vi "Move around TRAD v2.vi"() -> ()   [LabVIEW 2014]
uses:
  <vilib>/Instr/_visa.llb/VISA Configure Serial Port (Instr).vi
panel:
  in  "Numeric 2":i32
  in  "Short B desired":dbl
  in  "Short A desired":dbl
  in  "Move to position":bool
  in  "Home":bool
  out "number 2":i32
  out "number":i32
  in  "Dir":bool
  in  "Steps":u16(ring) items=["5", "10", "100", "1000", "10000"]
  in  "Move Tuner":bool
  in  "Save Position":bool
  in  "stop":bool
  in  "GO":bool
  in  "Change What":bool
  in  "Direction":bool
  out "Short B Value":dbl
  out "Short A Value":dbl
  out "Tuner Position":string
  # "Forward"
  # "Magnitude"
  # "Phase\nDifference"
  # "UP"
  # "Backward"
  # "DOWN"
  # "Move to a Particular Position"
  # "Go"
  # "Short B"
  # "Short A"
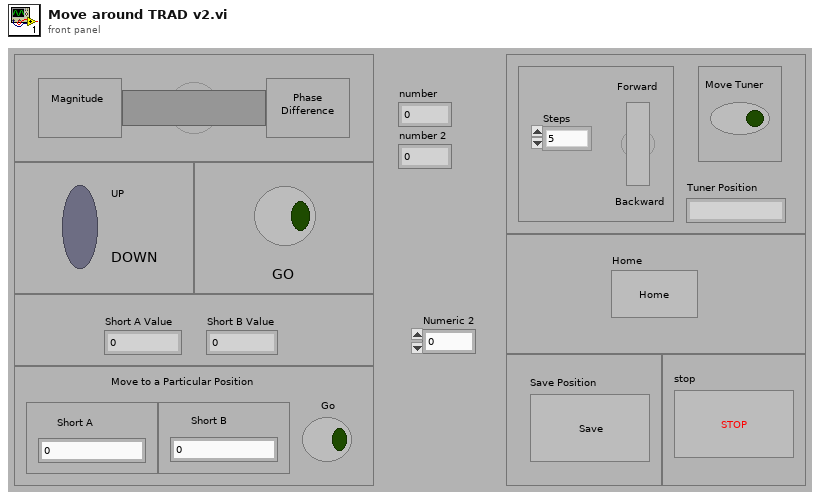
[diagram p1: front panel]
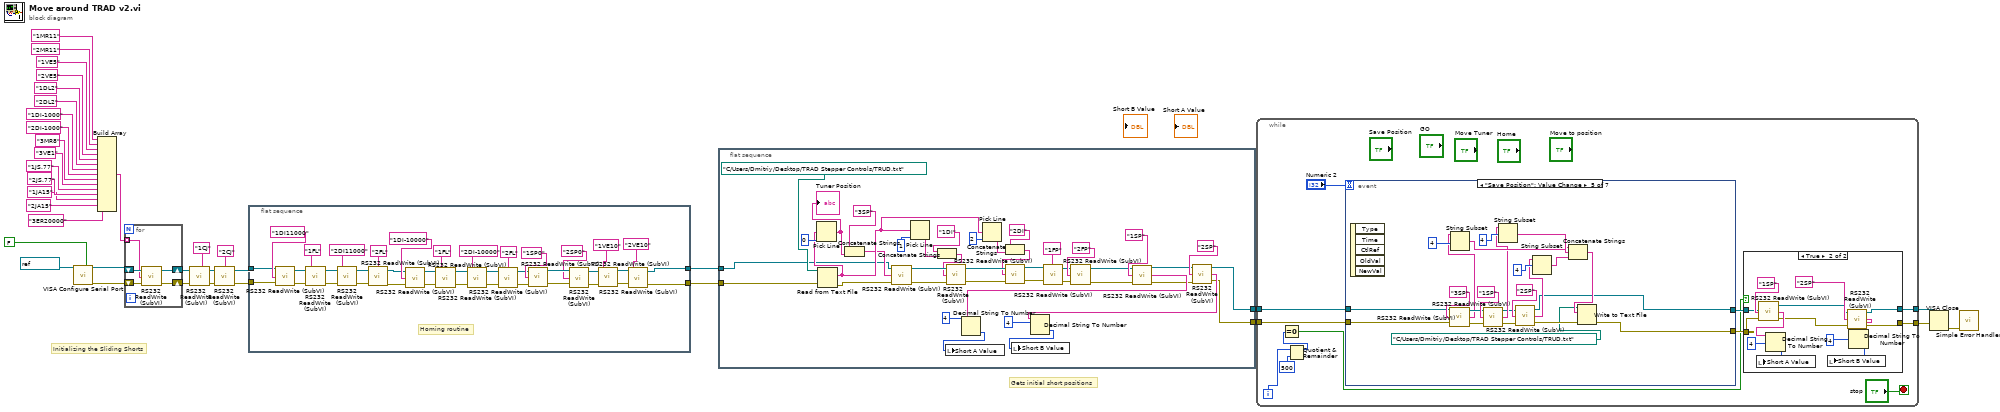
[diagram p0: block diagram]
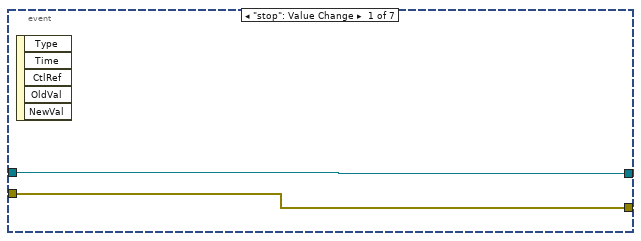
[diagram p3: hidden frame]
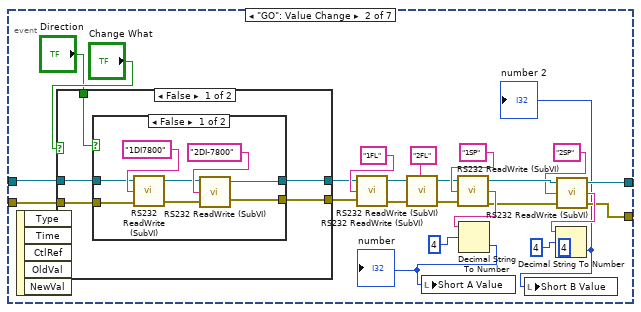
[diagram p4: hidden frame]
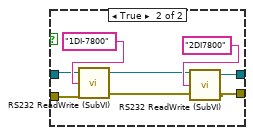
[diagram p5: hidden frame]
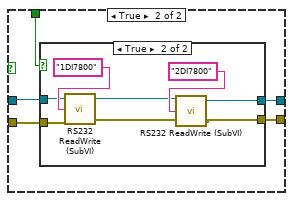
[diagram p6: hidden frame]
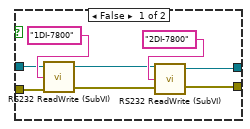
[diagram p7: hidden frame]
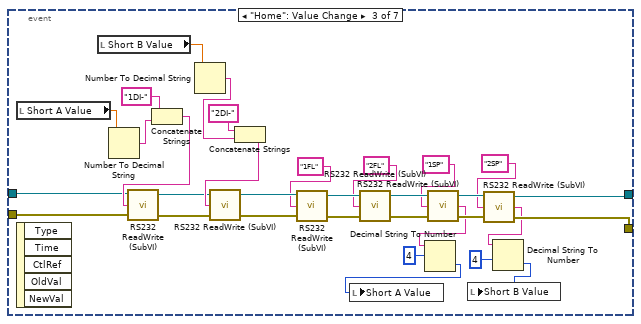
[diagram p8: hidden frame]
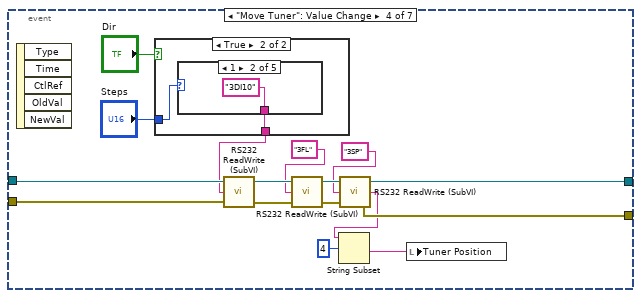
[diagram p9: hidden frame]
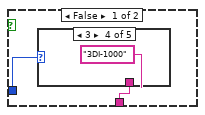
[diagram p10: hidden frame]
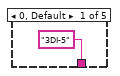
[diagram p11: hidden frame]
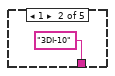
[diagram p12: hidden frame]
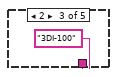
[diagram p13: hidden frame]
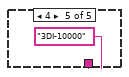
[diagram p14: hidden frame]
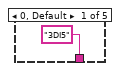
[diagram p15: hidden frame]
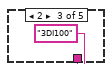
[diagram p16: hidden frame]
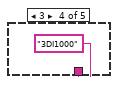
[diagram p17: hidden frame]
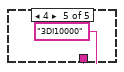
[diagram p18: hidden frame]
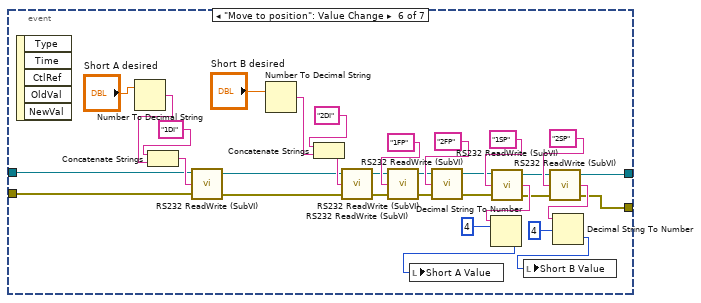
[diagram p19: hidden frame]
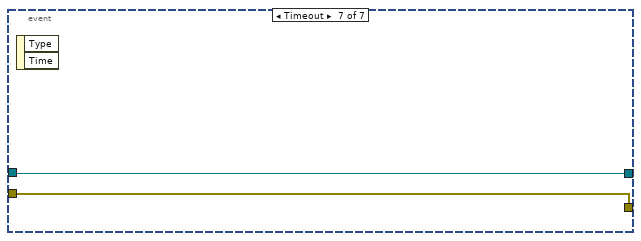
[diagram p20: hidden frame]
diagram:
  # "Initializing the Sliding Shorts"
  # "Gets initial short positions"
  n1 = call-poly "VISA Configure Serial Port"("VISA resource name"=refnum<visa-resource-name> "COM3", "Enable Termination\nChar (T)"=FALSE) -> ("VISA resource name out"=w18:refnum<visa-resource-name>, "error out"=w17:errorcluster)  [unwired: 12 in]
  n2 = Build Array("1MR11" ("Command to send to controller"), "2MR11" ("Command to send to controller"), "1VE5" ("Command to send to controller"), "2VE5" ("Command to send to controller"), "1DL2" ("Command to send to controller"), "2DL2" ("Command to send to controller"), "1DI-1000" ("Command to send to controller"), "2DI-1000" ("Command to send to controller"), "3MR8" ("Command to send to controller"), "3VE1" ("Command to send to controller"), "1JS.77", "2JS.77", "1JA15", "2JA15", "3ER20000") -> (w29:string[])
  n3 = for {
    shift-right: [w38] -> w15
    shift-left: w17 -> [w39]
    shift-right: [w37] -> w16
    shift-left: w18 -> [w40]
    tunnel: w29 -> [w36] mode=indexing
    n4 = call "RS232 ReadWrite (SubVI).vi"("error in (no error)"=w39, "Command to send to controller"=w36, "VISA resource name"=w40) -> ("error out"=w38:errorcluster, "VISA resource name out"=w37:refnum<visa-resource-name>)  [unwired: 1 out]
  }
  n5 = call "RS232 ReadWrite (SubVI).vi"("error in (no error)"=w15, "Command to send to controller"="1CJ", "VISA resource name"=w16) -> ("error out"=w6:errorcluster, "VISA resource name out"=w7:refnum<visa-resource-name>)  [unwired: 1 out]
  n6 = call "RS232 ReadWrite (SubVI).vi"("error in (no error)"=w6, "Command to send to controller"="2CJ", "VISA resource name"=w7) -> ("error out"=w13:errorcluster, "VISA resource name out"=w14:refnum<visa-resource-name>)  [unwired: 1 out]
  n7 = flat-sequence {
    tunnel: w13 -> [w63]
    tunnel: w14 -> [w64]
    tunnel: [w44] -> w4
    tunnel: [w43] -> w3
    frame #0 {
      # "Homing routine"
      n8 = call "RS232 ReadWrite (SubVI).vi"("error in (no error)"=w63, "Command to send to controller"="1DI11000", "VISA resource name"=w64) -> ("error out"=w75:errorcluster, "VISA resource name out"=w76:refnum<visa-resource-name>)  [unwired: 1 out]
      n9 = call "RS232 ReadWrite (SubVI).vi"("error in (no error)"=w75, "Command to send to controller"="1FL", "VISA resource name"=w76) -> ("error out"=w73:errorcluster, "VISA resource name out"=w74:refnum<visa-resource-name>)  [unwired: 1 out]
      n10 = call "RS232 ReadWrite (SubVI).vi"("error in (no error)"=w73, "Command to send to controller"="2DI11000", "VISA resource name"=w74) -> ("error out"=w71:errorcluster, "VISA resource name out"=w72:refnum<visa-resource-name>)  [unwired: 1 out]
      n11 = call "RS232 ReadWrite (SubVI).vi"("error in (no error)"=w71, "Command to send to controller"="2FL", "VISA resource name"=w72) -> ("error out"=w52:errorcluster, "VISA resource name out"=w51:refnum<visa-resource-name>)  [unwired: 1 out]
      n12 = call "RS232 ReadWrite (SubVI).vi"("error in (no error)"=w52, "Command to send to controller"="1DI-10000", "VISA resource name"=w51) -> ("error out"=w61:errorcluster, "VISA resource name out"=w62:refnum<visa-resource-name>)  [unwired: 1 out]
      n13 = call "RS232 ReadWrite (SubVI).vi"("error in (no error)"=w61, "Command to send to controller"="1FL", "VISA resource name"=w62) -> ("error out"=w59:errorcluster, "VISA resource name out"=w60:refnum<visa-resource-name>)  [unwired: 1 out]
      n14 = call "RS232 ReadWrite (SubVI).vi"("error in (no error)"=w59, "Command to send to controller"="2DI-10000", "VISA resource name"=w60) -> ("error out"=w57:errorcluster, "VISA resource name out"=w58:refnum<visa-resource-name>)  [unwired: 1 out]
      n15 = call "RS232 ReadWrite (SubVI).vi"("error in (no error)"=w57, "Command to send to controller"="2FL", "VISA resource name"=w58) -> ("error out"=w49:errorcluster, "VISA resource name out"=w50:refnum<visa-resource-name>)  [unwired: 1 out]
      n16 = call "RS232 ReadWrite (SubVI).vi"("error in (no error)"=w49, "Command to send to controller"="1SP0", "VISA resource name"=w50) -> ("error out"=w77:errorcluster, "VISA resource name out"=w78:refnum<visa-resource-name>)  [unwired: 1 out]
      n17 = call "RS232 ReadWrite (SubVI).vi"("error in (no error)"=w77, "Command to send to controller"="2SP0", "VISA resource name"=w78) -> ("error out"=w47:errorcluster, "VISA resource name out"=w48:refnum<visa-resource-name>)  [unwired: 1 out]
      n18 = call "RS232 ReadWrite (SubVI).vi"("error in (no error)"=w47, "Command to send to controller"="1VE10", "VISA resource name"=w48) -> ("error out"=w45:errorcluster, "VISA resource name out"=w46:refnum<visa-resource-name>)  [unwired: 1 out]
      n19 = call "RS232 ReadWrite (SubVI).vi"("error in (no error)"=w45, "Command to send to controller"="2VE10", "VISA resource name"=w46) -> ("error out"=w43:errorcluster, "VISA resource name out"=w44:refnum<visa-resource-name>)  [unwired: 1 out]
    }
  }
  n20 = flat-sequence {
    tunnel: [w82] -> w34
    tunnel: [w81] -> w2
    tunnel: w3 -> [w117]
    tunnel: w4 -> [w97]
    frame #0 {
      n21 = Read from Text File(file (use dialog)=path "C:/Users/Dmitriy/Desktop/TRAD Stepper Controls/TRUD.txt", error in=w117) -> (text=w115:string, error out=w112:errorcluster)  [unwired: 2 in, 2 out]
      n22 = Pick Line(multi-line string=w115, line index=0) -> (output string=w107:string)  [unwired: 1 in]
      "Tuner Position" <- w107
      n23 = Concatenate Strings("3SP" ("string"), w107) -> (w106:string)
      n24 = call "RS232 ReadWrite (SubVI).vi"("error in (no error)"=w112, "Command to send to controller"=w106, "VISA resource name"=w97) -> ("error out"=w113:errorcluster, "VISA resource name out"=w111:refnum<visa-resource-name>)  [unwired: 1 out]
      n25 = Pick Line(multi-line string=w115, line index=1) -> (output string=w101:string)  [unwired: 1 in]
      n26 = Concatenate Strings("1DI" ("string"), w101) -> (w103:string)
      n27 = call "RS232 ReadWrite (SubVI).vi"("error in (no error)"=w113, "Command to send to controller"=w103, "VISA resource name"=w111) -> ("error out"=w114:errorcluster, "VISA resource name out"=w110:refnum<visa-resource-name>)  [unwired: 1 out]
      n28 = Pick Line(multi-line string=w115, line index=2) -> (output string=w100:string)  [unwired: 1 in]
      n29 = Concatenate Strings("2DI" ("string"), w100) -> (w102:string)
      n30 = call "RS232 ReadWrite (SubVI).vi"("error in (no error)"=w114, "Command to send to controller"=w102, "VISA resource name"=w110) -> ("error out"=w93:errorcluster, "VISA resource name out"=w94:refnum<visa-resource-name>)  [unwired: 1 out]
      n31 = call "RS232 ReadWrite (SubVI).vi"("error in (no error)"=w93, "Command to send to controller"="1FP", "VISA resource name"=w94) -> ("error out"=w95:errorcluster, "VISA resource name out"=w92:refnum<visa-resource-name>)  [unwired: 1 out]
      n32 = call "RS232 ReadWrite (SubVI).vi"("error in (no error)"=w95, "Command to send to controller"="2FP", "VISA resource name"=w92) -> ("error out"=w79:errorcluster, "VISA resource name out"=w80:refnum<visa-resource-name>)  [unwired: 1 out]
      n33 = call "RS232 ReadWrite (SubVI).vi"("error in (no error)"=w79, "Command to send to controller"="1SP", "VISA resource name"=w80) -> ("error out"=w83:errorcluster, "String read from controller"=w87:string, "VISA resource name out"=w84:refnum<visa-resource-name>)
      n34 = Decimal String To Number(string=w87, offset=4) -> (number=w98:i32)  [unwired: 1 in, 1 out]
      n35 = local write "Short A Value"(w98) -> ()
      n36 = call "RS232 ReadWrite (SubVI).vi"("error in (no error)"=w83, "Command to send to controller"="2SP", "VISA resource name"=w84) -> ("error out"=w81:errorcluster, "String read from controller"=w88:string, "VISA resource name out"=w82:refnum<visa-resource-name>)
      n37 = Decimal String To Number(string=w88, offset=4) -> (number=w99:i32)  [unwired: 1 in, 1 out]
      n38 = local write "Short B Value"(w99) -> ()
    }
  }
  n39 = while {
    tunnel: w34 -> [w131]
    tunnel: [w122] -> w33
    tunnel: [w121] -> w32
    tunnel: w2 -> [w130]
    i -> [w126]
    stop <- "stop" stop-if-true
    n40 = Quotient & Remainder(x=w126, y=500) -> (x-y*floor(x/y)=w127:i32)  [unwired: 1 out]
    n41 = Equal To 0?(x=w127) -> (x = 0?=w120:bool)
    n42 = event shown="[4] \"Save Position\": Value Change" {
      selector: _ -> [_ _ _ _ _ _ _]
      dyn-events: _ -> [_ _ _ _ _ _ _]
      timeout: "Numeric 2" -> [_ _ _ _ _ _ _]
      tunnel: [w149 w159 w225 w257 w282 w306 w334] -> w124
      tunnel: w131 -> [w149 w153 w239 w262 w280 w326 w334]
      tunnel: w130 -> [w148 w152 w238 w263 w279 w325 w333]
      tunnel: [w148 w158 w224 w256 w281 w305 w333] -> w123
      event "stop": Value Change {
        n43 = event-data() -> ()  [unwired: 1 in, 5 out]
      }
      event "GO": Value Change {
        (unwired) 4
        n44 = event-data() -> ()  [unwired: 1 in, 5 out]
        n45 = case shown="False" "Change What" {
          tunnel: [w178 w199] -> w155
          tunnel: [w177 w198] -> w154
          tunnel: w153 -> [w176 w197]
          tunnel: w152 -> [w175 w196]
          tunnel: "Direction" -> [w174 w195]
          frame False {
            n46 = case shown="False" w174 {
              tunnel: [w182 w190] -> w178
              tunnel: [w181 w189] -> w177
              tunnel: w176 -> [w180 w188]
              tunnel: w175 -> [w179 w187]
              frame False {
                n47 = call "RS232 ReadWrite (SubVI).vi"("error in (no error)"=w179, "Command to send to controller"="1DI7800", "VISA resource name"=w180) -> ("error out"=w183:errorcluster, "VISA resource name out"=w184:refnum<visa-resource-name>)  [unwired: 1 out]
                n48 = call "RS232 ReadWrite (SubVI).vi"("error in (no error)"=w183, "Command to send to controller"="2DI-7800", "VISA resource name"=w184) -> ("error out"=w181:errorcluster, "VISA resource name out"=w182:refnum<visa-resource-name>)  [unwired: 1 out]
              }
              frame True {
                n49 = call "RS232 ReadWrite (SubVI).vi"("error in (no error)"=w187, "Command to send to controller"="1DI-7800", "VISA resource name"=w188) -> ("error out"=w191:errorcluster, "VISA resource name out"=w192:refnum<visa-resource-name>)  [unwired: 1 out]
                n50 = call "RS232 ReadWrite (SubVI).vi"("error in (no error)"=w191, "Command to send to controller"="2DI7800", "VISA resource name"=w192) -> ("error out"=w189:errorcluster, "VISA resource name out"=w190:refnum<visa-resource-name>)  [unwired: 1 out]
              }
            }
          }
          frame True {
            n51 = case shown="True" w195 {
              tunnel: [w203 w211] -> w199
              tunnel: [w202 w210] -> w198
              tunnel: w197 -> [w201 w209]
              tunnel: w196 -> [w200 w208]
              frame False {
                n52 = call "RS232 ReadWrite (SubVI).vi"("error in (no error)"=w200, "Command to send to controller"="1DI-7800", "VISA resource name"=w201) -> ("error out"=w204:errorcluster, "VISA resource name out"=w205:refnum<visa-resource-name>)  [unwired: 1 out]
                n53 = call "RS232 ReadWrite (SubVI).vi"("error in (no error)"=w204, "Command to send to controller"="2DI-7800", "VISA resource name"=w205) -> ("error out"=w202:errorcluster, "VISA resource name out"=w203:refnum<visa-resource-name>)  [unwired: 1 out]
              }
              frame True {
                n54 = call "RS232 ReadWrite (SubVI).vi"("error in (no error)"=w208, "Command to send to controller"="1DI7800", "VISA resource name"=w209) -> ("error out"=w212:errorcluster, "VISA resource name out"=w213:refnum<visa-resource-name>)  [unwired: 1 out]
                n55 = call "RS232 ReadWrite (SubVI).vi"("error in (no error)"=w212, "Command to send to controller"="2DI7800", "VISA resource name"=w213) -> ("error out"=w210:errorcluster, "VISA resource name out"=w211:refnum<visa-resource-name>)  [unwired: 1 out]
              }
            }
          }
        }
        n56 = call "RS232 ReadWrite (SubVI).vi"("error in (no error)"=w154, "Command to send to controller"="1FL", "VISA resource name"=w155) -> ("error out"=w170:errorcluster, "VISA resource name out"=w171:refnum<visa-resource-name>)  [unwired: 1 out]
        n57 = call "RS232 ReadWrite (SubVI).vi"("error in (no error)"=w170, "Command to send to controller"="2FL", "VISA resource name"=w171) -> ("error out"=w161:errorcluster, "VISA resource name out"=w160:refnum<visa-resource-name>)  [unwired: 1 out]
        n58 = call "RS232 ReadWrite (SubVI).vi"("error in (no error)"=w161, "Command to send to controller"="1SP", "VISA resource name"=w160) -> ("error out"=w165:errorcluster, "String read from controller"=w168:string, "VISA resource name out"=w166:refnum<visa-resource-name>)
        n59 = Decimal String To Number(string=w168, offset=4) -> (number=w157:i32)  [unwired: 1 in, 1 out]
        "number" <- w157
        n60 = local write "Short A Value"(w157) -> ()
        n61 = call "RS232 ReadWrite (SubVI).vi"("error in (no error)"=w165, "Command to send to controller"="2SP", "VISA resource name"=w166) -> ("error out"=w158:errorcluster, "String read from controller"=w164:string, "VISA resource name out"=w159:refnum<visa-resource-name>)
        n62 = Decimal String To Number(string=w164, offset=4 ("default (0 I32)")) -> (number=w156:i32)  [unwired: 1 in, 1 out]
        "number 2" <- w156
        n63 = local write "Short B Value"(w156) -> ()
      }
      event "Home": Value Change {
        n64 = local read "Short A Value"() -> (w245:dbl)
        n65 = event-data() -> ()  [unwired: 1 in, 5 out]
        n66 = local read "Short B Value"() -> (w240:dbl)
        n67 = Number To Decimal String(number=w245) -> (decimal integer string=w244:string)  [unwired: 1 in]
        n68 = Concatenate Strings("1DI-" ("string"), w244) -> (w243:string)
        n69 = call "RS232 ReadWrite (SubVI).vi"("error in (no error)"=w238, "Command to send to controller"=w243, "VISA resource name"=w239) -> ("error out"=w236:errorcluster, "VISA resource name out"=w237:refnum<visa-resource-name>)  [unwired: 1 out]
        n70 = Number To Decimal String(number=w240) -> (decimal integer string=w242:string)  [unwired: 1 in]
        n71 = Concatenate Strings("2DI-" ("string"), w242) -> (w241:string)
        n72 = call "RS232 ReadWrite (SubVI).vi"("error in (no error)"=w236, "Command to send to controller"=w241, "VISA resource name"=w237) -> ("error out"=w234:errorcluster, "VISA resource name out"=w235:refnum<visa-resource-name>)  [unwired: 1 out]
        n73 = call "RS232 ReadWrite (SubVI).vi"("error in (no error)"=w234, "Command to send to controller"="1FL", "VISA resource name"=w235) -> ("error out"=w232:errorcluster, "VISA resource name out"=w233:refnum<visa-resource-name>)  [unwired: 1 out]
        n74 = call "RS232 ReadWrite (SubVI).vi"("error in (no error)"=w232, "Command to send to controller"="2FL", "VISA resource name"=w233) -> ("error out"=w228:errorcluster, "VISA resource name out"=w229:refnum<visa-resource-name>)  [unwired: 1 out]
        n75 = call "RS232 ReadWrite (SubVI).vi"("error in (no error)"=w228, "Command to send to controller"="1SP", "VISA resource name"=w229) -> ("error out"=w227:errorcluster, "String read from controller"=w220:string, "VISA resource name out"=w226:refnum<visa-resource-name>)
        n76 = Decimal String To Number(string=w220, offset=4 ("offset (0)")) -> (number=w217:i32)  [unwired: 1 in, 1 out]
        n77 = local write "Short A Value"(w217) -> ()
        n78 = call "RS232 ReadWrite (SubVI).vi"("error in (no error)"=w227, "Command to send to controller"="2SP", "VISA resource name"=w226) -> ("error out"=w224:errorcluster, "String read from controller"=w221:string, "VISA resource name out"=w225:refnum<visa-resource-name>)
        n79 = Decimal String To Number(string=w221, offset=4 ("offset (0)")) -> (number=w218:i32)  [unwired: 1 in, 1 out]
        n80 = local write "Short B Value"(w218) -> ()
      }
      event "Move Tuner": Value Change {
        n81 = event-data() -> ()  [unwired: 1 in, 5 out]
        n82 = case shown="True" "Dir" {
          tunnel: "Steps" -> [w265 w272]
          tunnel: [w264 w271] -> w250
          frame False {
            n83 = case shown="3" w265 {
              tunnel: ["3DI-5" "3DI-10" "3DI-100" "3DI-1000" "3DI-10000"] -> w264
              frame 0, Default {
              }
              frame 1 {
              }
              frame 2 {
              }
              frame 3 {
              }
              frame 4 {
              }
            }
          }
          frame True {
            n84 = case shown="1" w272 {
              tunnel: ["3DI5" "3DI10" "3DI100" "3DI1000" "3DI10000"] -> w271
              frame 0, Default {
              }
              frame 1 {
              }
              frame 2 {
              }
              frame 3 {
              }
              frame 4 {
              }
            }
          }
        }
        n85 = call "RS232 ReadWrite (SubVI).vi"("error in (no error)"=w263, "Command to send to controller"=w250, "VISA resource name"=w262) -> ("error out"=w260:errorcluster, "VISA resource name out"=w261:refnum<visa-resource-name>)  [unwired: 1 out]
        n86 = call "RS232 ReadWrite (SubVI).vi"("error in (no error)"=w260, "Command to send to controller"="3FL", "VISA resource name"=w261) -> ("error out"=w258:errorcluster, "VISA resource name out"=w259:refnum<visa-resource-name>)  [unwired: 1 out]
        n87 = call "RS232 ReadWrite (SubVI).vi"("error in (no error)"=w258, "Command to send to controller"="3SP", "VISA resource name"=w259) -> ("error out"=w256:errorcluster, "String read from controller"=w253:string, "VISA resource name out"=w257:refnum<visa-resource-name>)
        n88 = String Subset(string=w253, offset (0)=4) -> (substring=w251:string)  [unwired: 1 in]
        n89 = local write "Tuner Position"(w251) -> ()
      }
      event "Save Position": Value Change {
        n90 = event-data() -> ()  [unwired: 1 in, 5 out]
        n91 = call "RS232 ReadWrite (SubVI).vi"("error in (no error)"=w279, "Command to send to controller"="3SP", "VISA resource name"=w280) -> ("error out"=w286:errorcluster, "String read from controller"=w284:string, "VISA resource name out"=w289:refnum<visa-resource-name>)
        n92 = String Subset(string=w284, offset (0)=4) -> (substring=w297:string)  [unwired: 1 in]
        n93 = call "RS232 ReadWrite (SubVI).vi"("error in (no error)"=w286, "Command to send to controller"="1SP", "VISA resource name"=w289) -> ("error out"=w287:errorcluster, "String read from controller"=w294:string, "VISA resource name out"=w290:refnum<visa-resource-name>)
        n94 = String Subset(string=w294, offset (0)=4) -> (substring=w299:string)  [unwired: 1 in]
        n95 = call "RS232 ReadWrite (SubVI).vi"("error in (no error)"=w287, "Command to send to controller"="2SP", "VISA resource name"=w290) -> ("error out"=w288:errorcluster, "String read from controller"=w293:string, "VISA resource name out"=w282:refnum<visa-resource-name>)
        n96 = String Subset(string=w293, offset (0)=4) -> (substring=w300:string)  [unwired: 1 in]
        n97 = Concatenate Strings(w297, w299, w300) -> (w298:string)
        n98 = Write to Text File(file (use dialog)=path "C:/Users/Dmitriy/Desktop/TRAD Stepper Controls/TRUD.txt", text=w298, error in=w288) -> (error out=w281:errorcluster)  [unwired: 1 in, 2 out]
      }
      event "Move to position": Value Change {
        n99 = event-data() -> ()  [unwired: 1 in, 5 out]
        n100 = Number To Decimal String(number="Short A desired") -> (decimal integer string=w329:string)  [unwired: 1 in]
        n101 = Concatenate Strings("1DI" ("string"), w329) -> (w328:string)
        n102 = call "RS232 ReadWrite (SubVI).vi"("error in (no error)"=w325, "Command to send to controller"=w328, "VISA resource name"=w326) -> ("error out"=w323:errorcluster, "VISA resource name out"=w324:refnum<visa-resource-name>)  [unwired: 1 out]
        n103 = Number To Decimal String(number="Short B desired") -> (decimal integer string=w330:string)  [unwired: 1 in]
        n104 = Concatenate Strings("2DI" ("string"), w330) -> (w327:string)
        n105 = call "RS232 ReadWrite (SubVI).vi"("error in (no error)"=w323, "Command to send to controller"=w327, "VISA resource name"=w324) -> ("error out"=w319:errorcluster, "VISA resource name out"=w320:refnum<visa-resource-name>)  [unwired: 1 out]
        n106 = call "RS232 ReadWrite (SubVI).vi"("error in (no error)"=w319, "Command to send to controller"="1FP", "VISA resource name"=w320) -> ("error out"=w318:errorcluster, "VISA resource name out"=w317:refnum<visa-resource-name>)  [unwired: 1 out]
        n107 = call "RS232 ReadWrite (SubVI).vi"("error in (no error)"=w318, "Command to send to controller"="2FP", "VISA resource name"=w317) -> ("error out"=w308:errorcluster, "VISA resource name out"=w307:refnum<visa-resource-name>)  [unwired: 1 out]
        n108 = call "RS232 ReadWrite (SubVI).vi"("error in (no error)"=w308, "Command to send to controller"="1SP", "VISA resource name"=w307) -> ("error out"=w309:errorcluster, "String read from controller"=w314:string, "VISA resource name out"=w310:refnum<visa-resource-name>)
        n109 = Decimal String To Number(string=w314, offset=4 ("offset (0)")) -> (number=w303:i32)  [unwired: 1 in, 1 out]
        n110 = local write "Short A Value"(w303) -> ()
        n111 = call "RS232 ReadWrite (SubVI).vi"("error in (no error)"=w309, "Command to send to controller"="2SP", "VISA resource name"=w310) -> ("error out"=w305:errorcluster, "String read from controller"=w313:string, "VISA resource name out"=w306:refnum<visa-resource-name>)
        n112 = Decimal String To Number(string=w313, offset=4 ("offset (0)")) -> (number=w304:i32)  [unwired: 1 in, 1 out]
        n113 = local write "Short B Value"(w304) -> ()
      }
      event Timeout {
        n114 = event-data() -> ()  [unwired: 1 in, 2 out]
      }
    }
    n115 = case shown="True" w120 {
      tunnel: w124 -> [w132 w139]
      tunnel: w123 -> [w133 w136]
      tunnel: [w132 w138] -> w122
      tunnel: [w133 w137] -> w121
      frame False {
      }
      frame True {
        n116 = call "RS232 ReadWrite (SubVI).vi"("error in (no error)"=w136, "Command to send to controller"="1SP", "VISA resource name"=w139) -> ("error out"=w140:errorcluster, "String read from controller"=w145:string, "VISA resource name out"=w141:refnum<visa-resource-name>)
        n117 = Decimal String To Number(string=w145, offset=4 ("offset (0)")) -> (number=w134:i32)  [unwired: 1 in, 1 out]
        n118 = local write "Short A Value"(w134) -> ()
        n119 = call "RS232 ReadWrite (SubVI).vi"("error in (no error)"=w140, "Command to send to controller"="2SP", "VISA resource name"=w141) -> ("error out"=w137:errorcluster, "String read from controller"=w144:string, "VISA resource name out"=w138:refnum<visa-resource-name>)
        n120 = Decimal String To Number(string=w144, offset=4 ("offset (0)")) -> (number=w135:i32)  [unwired: 1 in, 1 out]
        n121 = local write "Short B Value"(w135) -> ()
      }
    }
  }
  n122 = VISA Close(VISA resource name=w33, error in (no error)=w32) -> (error out=w35:errorcluster)
  n123 = call <vilib>:"Simple Error Handler.vi"("error in (no error)"=w35) -> ()  [unwired: 4 in, 5 out]
